vi "Write Active Channel.vi"(8 "error in":errorcluster, 10 "Active Channel":T1, 11 "Power Supply in":refnum<class "Power Supply.lvclass">) -> (0 "error out":errorcluster, 3 "Power Supply out":refnum<class "Power Supply.lvclass">)   [LabVIEW 2018, in "Power Supply.lvlib" / "Power Supply.lvclass"]
uses:
  Power Supply.lvclass
  Custom Control/Channel List.ctl
  Power Supply.lvclass/Power Supply.ctl
  Power Supply.lvlib
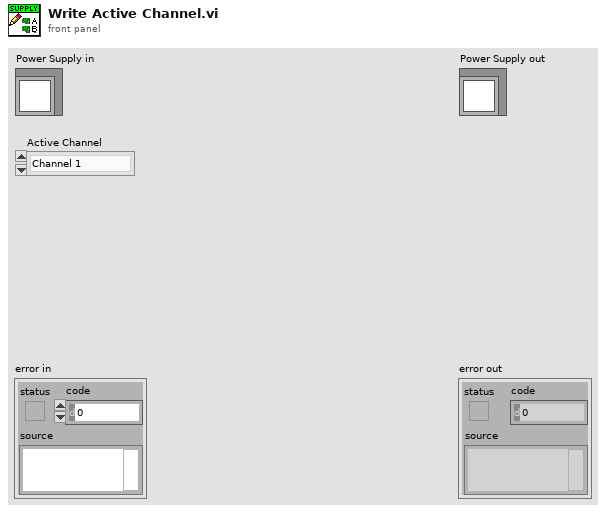
[diagram p1: front panel]
types:
  T1 = typedef "Power Supply.lvlib/Channel List.ctl" = enum16{"Channel 1", "Channel 2", "Channel 3", "Channel 4"}
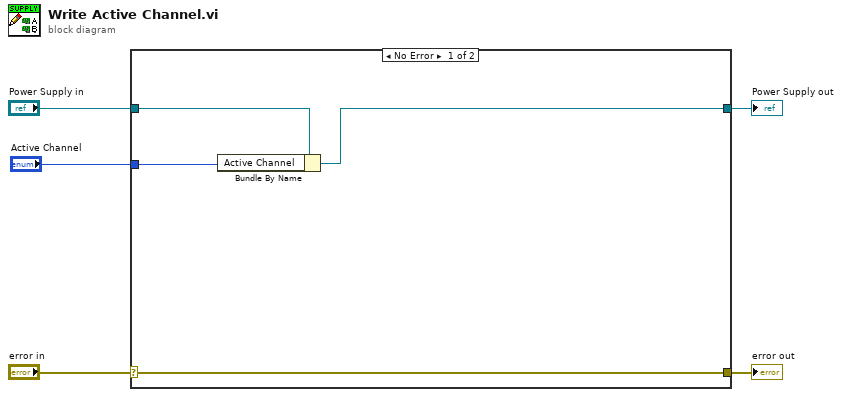
[diagram p0: block diagram]
diagram:
  n1 = case shown="No Error" "error in" {
    selector: "error in" -> [w8 w11]
    tunnel: [w8 w11] -> w4
    tunnel: [w7 w10] -> w2
    tunnel: "Power Supply in" -> [w9 w10]
    tunnel: "Active Channel" -> [w6 _]
    frame No Error {
      n2 = Bundle By Name(cluster=w9, "Active Channel"=w6) -> (w7:refnum<class "Power Supply.lvclass">)
    }
    frame Error {
    }
  }
  "error out" <- w4
  "Power Supply out" <- w2
